vi "Yokogawa WT1800 Series Acquire Continuous Waveform.vi"() -> ()   [LabVIEW 2015]
doc: "This example shows how to use auto ranging and acquire a waveform on a single trace."
uses:
  <instrlib>/Yokogawa WT1800 Series/Public/Configure/Configure Range (Voltage).vi
  <instrlib>/Yokogawa WT1800 Series/Public/Configure/Configure Range (Current 50A).vi
  <instrlib>/Yokogawa WT1800 Series/Public/Data/Read Waveform (Single).vi
  <instrlib>/Yokogawa WT1800 Series/Yokogawa WT1800 Series.lvlib
panel:
  in  "Update Rate (500ms)":dbl(ring)=0.5 items=["50m"=0.05, "100m"=0.1, "200m"=0.2, "500m"=0.5, "1"=1.0, "2"=2.0, "5"=5.0, "10"=10.0, "20"=20.0]
  in  "stop":bool
  in  "Auto Range (F: Disable)":bool
  in  "Trace (0: U1)":i32(ring) items=["U1", "I1", "U2", "I2", "U3", "I3", "U4", "I4", "U5", "I5", "U6", "I6", "Speed", "Torque", "AUX1", "AUX2"]
  in  "Timeout (10000 ms)":i32=10000 min=1
  in  "VISA resource name":refnum<visa-resource-name>
  out "Waveform Graph":T1(graph)
  # "(c) 2011 Yokogawa Meters & Instruments Corporation.  All rights reserved."
  # "WT1800 SERIES POWER ANALYZER"
  # "s"
  # "ms"
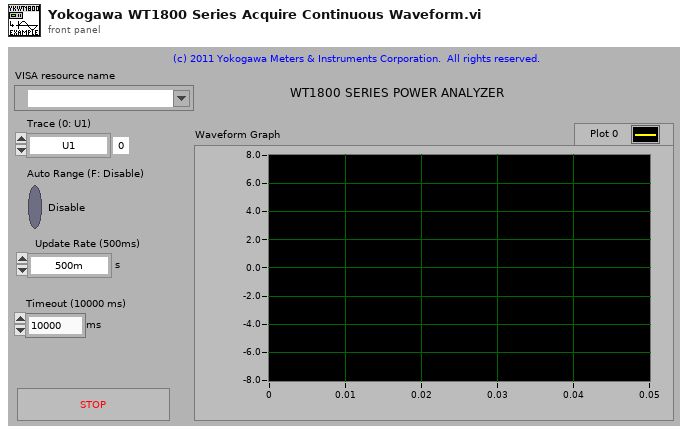
[diagram p1: front panel]
types:
  T1 = cluster{"start":dbl, "Sampling Time":dbl, "Output":dbl[]}
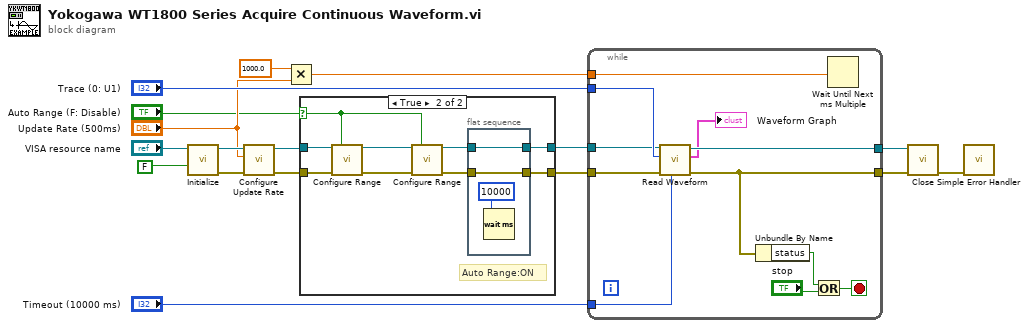
[diagram p0: block diagram]
diagram:
  n1 = call <instrlib>:"Initialize.vi"("Reset (True)"=FALSE, "VISA resource name"="VISA resource name") -> ("error out"=w7:errorcluster, "VISA resource name out"=w8:refnum<visa-resource-name>)  [unwired: 8 in]
  n2 = call <instrlib>:"Configure Update Rate.vi"("error in (no error)"=w7, "Update Rate (500m s)"="Update Rate (500ms)", "VISA resource name"=w8) -> ("error out"=w3:errorcluster, "VISA resource name out"=w4:refnum<visa-resource-name>)  [unwired: 7 in]
  n3 = Multiply(x=1000.0, y="Update Rate (500ms)") -> (x*y=w1:dbl)
  n4 = case shown="True" "Auto Range (F: Disable)" {
    selector: "Auto Range (F: Disable)" -> [_ w20]
    tunnel: w3 -> [w18 w23]
    tunnel: [w18 w28] -> w11
    tunnel: w4 -> [w19 w24]
    tunnel: [w19 w27] -> w10
    frame False {
      # "Auto Range:OFF"
    }
    frame True {
      # "Auto Range:ON"
      n5 = call-poly <instrlib>:"Configure Range.vi"("VISA resource name"=w24, "Auto Range (F: Disable)"=w20, "error in (no error)"=w23) -> ("VISA resource name out"=w25:refnum<visa-resource-name>, "error out"=w26:errorcluster)  [unwired: 11 in]
      n6 = call-poly <instrlib>:"Configure Range.vi"("VISA resource name"=w25, "Auto Range (F: Disable)"=w20, "error in (no error)"=w26) -> ("VISA resource name out"=w22:refnum<visa-resource-name>, "error out"=w21:errorcluster)  [unwired: 11 in]
      n7 = flat-sequence {
        tunnel: [w30] -> w28
        tunnel: w21 -> [w30]
        tunnel: [w29] -> w27
        tunnel: w22 -> [w29]
        frame #0 {
          n8 = Wait (ms)(milliseconds to wait=u32 10000 ("ミリ秒待ち時間")) -> ()  [unwired: 1 out]
        }
      }
    }
  }
  n9 = while {
    tunnel: "Trace (0: U1)" -> [w42]
    tunnel: [w41] -> w14
    tunnel: [w33] -> w13
    tunnel: w11 -> [w39]
    tunnel: w10 -> [w38]
    tunnel: "Timeout (10000 ms)" -> [w37]
    tunnel: w1 -> [w32]
    stop <- w34 stop-if-true
    n10 = call-poly <instrlib>:"Read Waveform.vi"("Timeout (10000 ms)"=w37, "error in (no error)"=w39, "Trace (0: U1)"=w42, "VISA resource name"=w38) -> ("error out"=w33:errorcluster, "Waveform Data"=→"Waveform Graph":T1, "VISA resource name out"=w41:refnum<visa-resource-name>)  [unwired: 5 in]
    n11 = Unbundle By Name ("名前でバンドル解除")(w33) -> ("status"=w36:bool)
    n12 = Or(x=w36, y="stop") -> (x .or. y?=w34:bool)
    n13 = Wait Until Next ms Multiple(millisecond multiple=w32) -> ()  [unwired: 1 out]
  }
  n14 = call <instrlib>:"Close.vi"("error in (no error)"=w13, "VISA resource name"=w14) -> ("error out"=w12:errorcluster)  [unwired: 9 in]
  n15 = call <vilib>:"Simple Error Handler.vi"("error in (no error)"=w12) -> ()  [unwired: 4 in, 5 out]
